vi "PickPlace.vi"(4 "controller":refnum<k24>, 5 "Tool or Plate":enum16{"Tool", "Plate"}(ring), 6 "error in (no error)":errorcluster, 7 "Pick or Drop":enum16{"Pick", "Drop"}(ring)) -> (0 "error out":errorcluster, 2 "controller out":refnum<k24>, 3 "sensor on?":bool)   [LabVIEW 2019]
uses:
  C:/Users/TTUHEP/Documents/LabVIEW/Other Models/2010/Bin/Aerotech.A3200.dll
  Other Models/2010/Bin/Aerotech.A3200.dll
  Other Models/2010/Motion/AbortSingle.vi
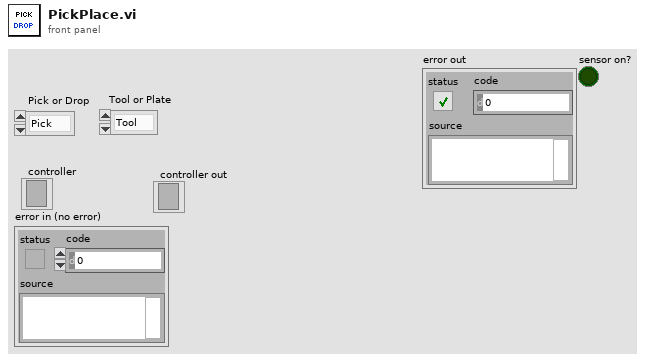
[diagram p1: front panel]
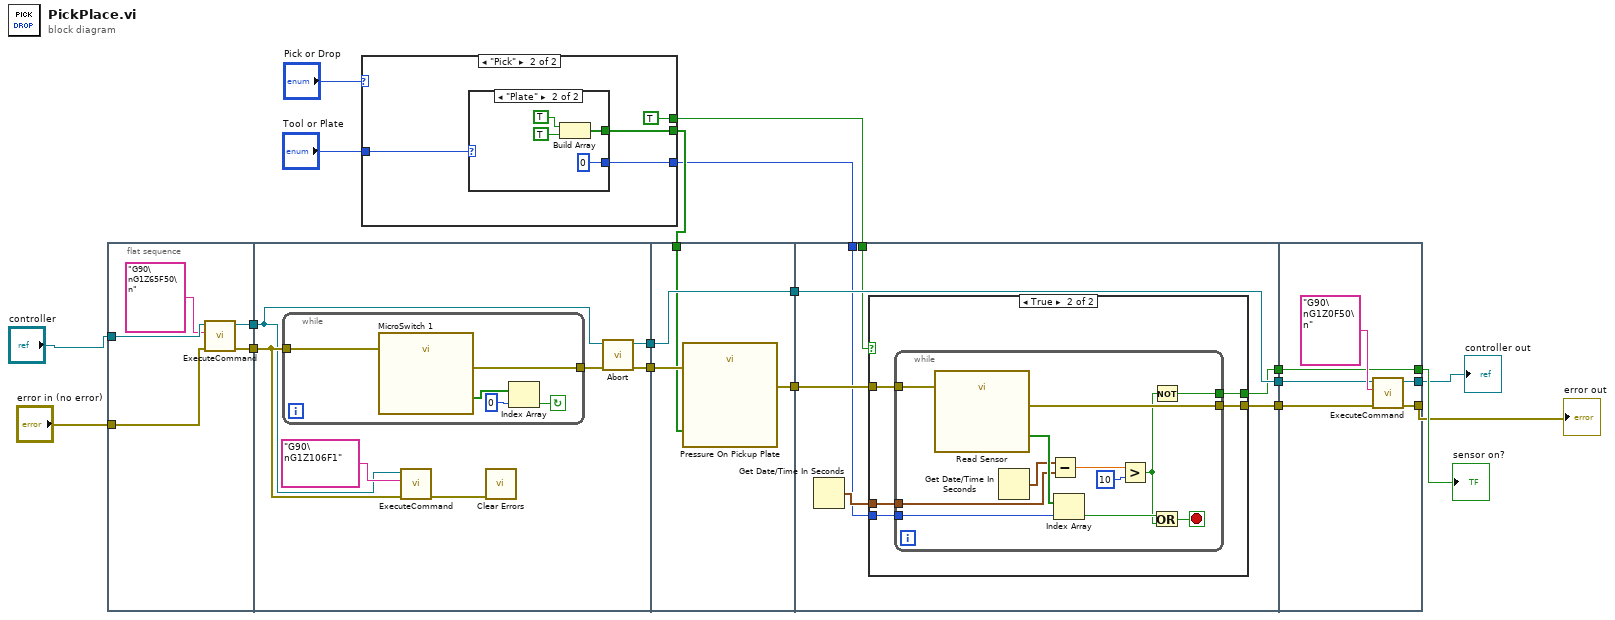
[diagram p0: block diagram]
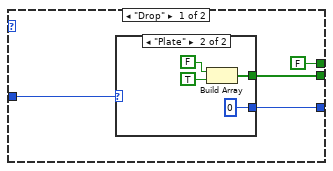
[diagram p2: hidden frame]
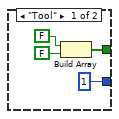
[diagram p3: hidden frame]
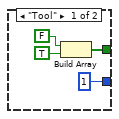
[diagram p4: hidden frame]
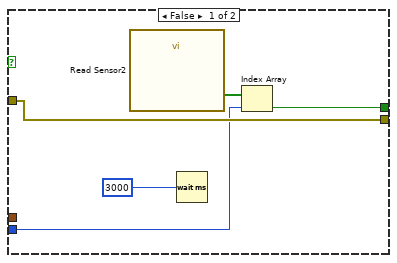
[diagram p5: hidden frame]
diagram:
  n1 = flat-sequence {
    tunnel: "controller" -> [w24]
    tunnel: [w23] -> w19
    tunnel: [w22] -> w18
    tunnel: "error in (no error)" -> [w20]
    tunnel: w19 -> [w27]
    tunnel: w18 -> [w30]
    tunnel: [w28] -> w17
    tunnel: [w26] -> w16
    tunnel: w17 -> [w40]
    tunnel: w16 -> [w39]
    tunnel: [w40] -> w15
    tunnel: [w38] -> w14
    tunnel: w9 -> [w37]
    tunnel: w15 -> [w47]
    tunnel: w14 -> [w46]
    tunnel: [w47] -> w13
    tunnel: [w44] -> w12
    tunnel: [w43] -> w10
    tunnel: w8 -> [w42]
    tunnel: w7 -> [w41]
    tunnel: w13 -> [w73]
    tunnel: w12 -> [w74]
    tunnel: [w72] -> w1
    tunnel: [w71] -> w2
    tunnel: [w70] -> w11
    tunnel: w10 -> [w70]
    frame #0 {
      n2 = call "ExecuteCommand.vi"("error in (no error)"=w20, "Command Code"="G90\nG1Z65F50\n", "controller in"=w24) -> ("error out"=w22:errorcluster, "controller out"=w23:refnum<k24>)  [unwired: 6 in, 1 out]
    }
    frame #1 {
      n3 = while {
        tunnel: [w36] -> w29
        tunnel: w30 -> [w35]
        stop <- w33 continue-if-true
        n4 = call "MicroSwitch 1"("error in"=w35) -> ("data"=w34:bool[], "error out"=w36:errorcluster)  [unwired: 16 in, 1 out]
        n5 = Index Array(array=w34, index=0) -> (element=w33:bool)
      }
      n6 = call "ExecuteCommand.vi"("error in (no error)"=w30, "Command Code"="G90\nG1Z106F1", "controller in"=w27) -> ("error out"=w25:errorcluster)  [unwired: 6 in, 2 out]
      n7 = call <vilib>:"Clear Errors.vi"("error in (no error)"=w25) -> ()  [unwired: 5 in, 2 out]
      n8 = call-poly "Abort.vi"("error in (no error)"=w29, "controller in"=w27) -> ("error out"=w26:errorcluster, "controller out"=w28:refnum<k24>)  [unwired: 8 in]
    }
    frame #2 {
      n9 = call "Pressure On Pickup Plate"("data"=w37, "error in"=w39) -> ("error out"=w38:errorcluster)  [unwired: 16 in, 1 out]
    }
    frame #3 {
      n10 = Get Date/Time In Seconds() -> (seconds since 1Jan1904=w45:timestamp)
      n11 = case shown="True" w41 {
        tunnel: w46 -> [w52 w57]
        tunnel: w45 -> [_ w56]
        tunnel: [w52 w55] -> w44
        tunnel: [w49 w54] -> w43
        tunnel: w42 -> [w50 w53]
        frame False {
          n12 = call "Read Sensor2"() -> ("data"=w51:bool[])  [unwired: 17 in, 2 out]
          n13 = Wait (ms)(milliseconds to wait=3000) -> ()  [unwired: 1 out]
          n14 = Index Array(array=w51, index=w50) -> (element=w49:bool)
        }
        frame True {
          n15 = while {
            tunnel: w57 -> [w68]
            tunnel: w56 -> [w64]
            tunnel: [w62] -> w55
            tunnel: [w61] -> w54
            tunnel: w53 -> [w60]
            stop <- w63 stop-if-true
            n16 = call "Read Sensor"("error in"=w68) -> ("data"=w69:bool[], "error out"=w62:errorcluster)  [unwired: 16 in, 1 out]
            n17 = Get Date/Time In Seconds() -> (seconds since 1Jan1904=w67:timestamp)
            n18 = Subtract(x=w67, y=w64) -> (x-y=w65:dbl)
            n19 = Index Array(array=w69, index=w60) -> (element=w59:bool)
            n20 = Greater?(x=w65, y=10) -> (0:w58:bool)
            n21 = Not(x=w58) -> (.not. x?=w61:bool)
            n22 = Or(x=w59, y=w58) -> (x .or. y?=w63:bool)
          }
        }
      }
    }
    frame #4 {
      n23 = call "ExecuteCommand.vi"("error in (no error)"=w74, "Command Code"="G90\nG1Z0F50\n", "controller in"=w73) -> ("error out"=w71:errorcluster, "controller out"=w72:refnum<k24>)  [unwired: 6 in, 1 out]
    }
  }
  n24 = case shown="\"Pick\"" "Pick or Drop" {
    tunnel: "Tool or Plate" -> [w76 w91]
    tunnel: [w79 w90] -> w9
    tunnel: [w78 w89] -> w8
    tunnel: [FALSE TRUE] -> w7
    frame "Drop" {
      n25 = case shown="\"Plate\"" w76 {
        tunnel: [w81 w85] -> w79
        tunnel: [1 0] -> w78
        frame "Tool" {
          n26 = Build Array(FALSE, FALSE) -> (w81:bool[])
        }
        frame "Plate" {
          n27 = Build Array(FALSE, TRUE) -> (w85:bool[])
        }
      }
    }
    frame "Pick" {
      n28 = case shown="\"Plate\"" w91 {
        tunnel: [w93 w97] -> w90
        tunnel: [1 0] -> w89
        frame "Tool" {
          n29 = Build Array(FALSE, TRUE) -> (w93:bool[])
        }
        frame "Plate" {
          n30 = Build Array(TRUE, TRUE) -> (w97:bool[])
        }
      }
    }
  }
  "error out" <- w2
  "sensor on?" <- w11
  "controller out" <- w1
